vi "DB Tools Create Table If Not Exist.vi"(4 "parameters":T1[](array[typedef]), 5 "use file? (F)":bool, 6 "error in (no error)":errorcluster, 7 "columns":string[](array[string]), 8 "table name":string, 9 "connection reference":T4) -> (0 "error out":errorcluster, 1 "columns out":string[](array[string]), 2 "table name out":string, 3 "connection reference out":T4)   [LabVIEW 2012, in "NI_Database_API_64.lvlib"]
doc: "Creates a new table in the database identified by <B>connection reference</B> if that table does not already exist. The <B>table name</B>, <B>columns</B>, and <B>parameters</B> inputs describe the name of the table, the names of the columns (fields), and the parameter properties of each column, respectively."
uses:
  NI_Database_API_64.lvlib
  Connection.llb/Conn ObjectReference.ctl
  DB Tools Parameter Info.ctl
  DB Tools DataTypes.ctl
  DB Tools Parameter Dir.ctl
  DB Tools Column Info.ctl
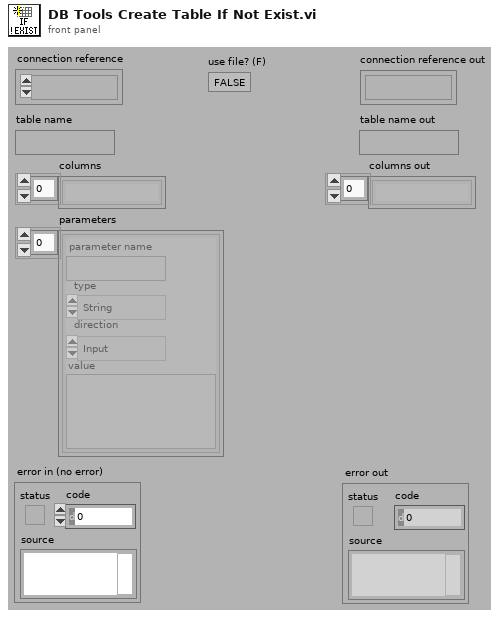
[diagram p1: front panel]
types:
  T1 = typedef "NI_Database_API_64.lvlib/DB Tools Parameter Info.ctl" = cluster{"parameter name":string, "type":T2, "direction":T3, "value":variant}
  T2 = typedef "NI_Database_API_64.lvlib/DB Tools DataTypes.ctl" = enum16{"String", "Long (I32)", "Single (SGL)", "Double (DBL)", "Date/Time", "Binary"}
  T3 = typedef "NI_Database_API_64.lvlib/DB Tools Parameter Dir.ctl" = enum32{"Input", "Output", "Input/Output", "Return Value"}
  T4 = typedef "NI_Database_API_64.lvlib/Conn ObjectReference.ctl" = refnum<k1>
  T5 = typedef "NI_Database_API_64.lvlib/DB Tools Column Info.ctl" = cluster{"column name":string, "data type":T2, "size":i32, "allow null?":bool}
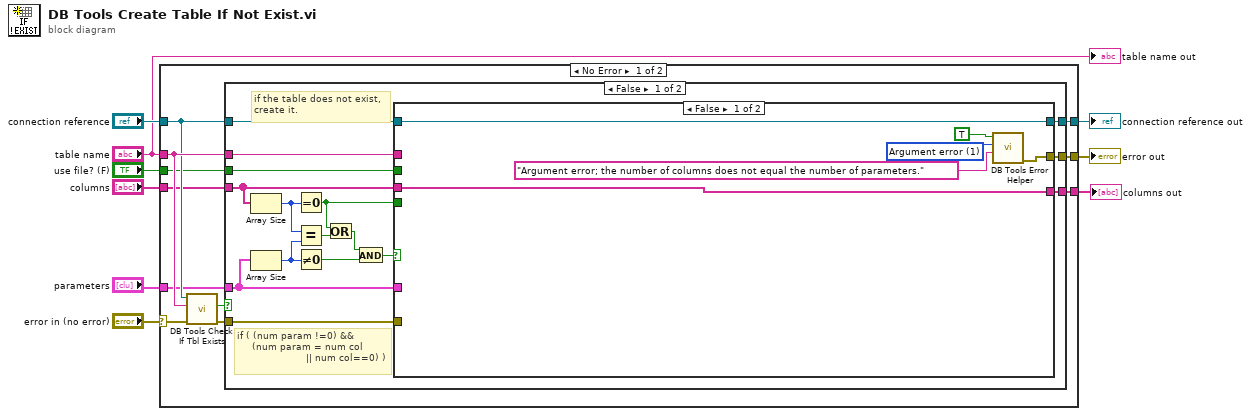
[diagram p0: block diagram]
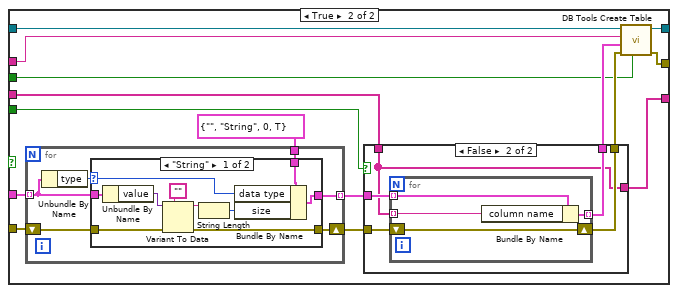
[diagram p2: hidden frame]
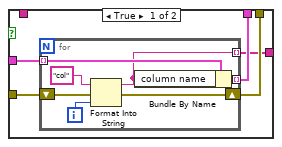
[diagram p3: hidden frame]
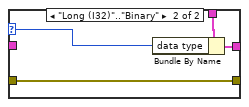
[diagram p4: hidden frame]
diagram:
  n1 = case shown="No Error" "error in (no error)" {
    selector: "error in (no error)" -> [w10 w104]
    tunnel: "connection reference" -> [w15 w103]
    tunnel: "table name" -> [w18 _]
    tunnel: [w17 w104] -> w7
    tunnel: [w16 w103] -> w6
    tunnel: "columns" -> [w14 w102]
    tunnel: "parameters" -> [w12 _]
    tunnel: [w13 w102] -> w3
    tunnel: "use file? (F)" -> [w11 _]
    frame No Error {
      n2 = call "DB Tools Check If Tbl Exists.vi"("error in (no error)"=w10, "table name"=w18, "connection reference"=w15) -> ("error out"=w20:errorcluster, "exists?"=w19:bool)  [unwired: 3 out]
      n3 = case shown="False" w19 {
        tunnel: w20 -> [w26 w101]
        tunnel: w18 -> [w36 _]
        tunnel: [w35 w101] -> w17
        tunnel: [w34 w100] -> w16
        tunnel: w15 -> [w33 w100]
        tunnel: w14 -> [w28 w99]
        tunnel: w12 -> [w22 _]
        tunnel: [w24 w99] -> w13
        tunnel: w11 -> [w21 _]
        frame False {
          # "if ( (num param !=0) &&\n     (num param = num col \n                       || num col==0) )"
          # "if the table does not exist, \ncreate it."
          n4 = Array Size(array=w28) -> (size(s)=w32:i32)
          n5 = Array Size(array=w22) -> (size(s)=w25:i32)
          n6 = Equal To 0?(x=w32) -> (x = 0?=w23:bool)
          n7 = Equal?(x=w32, y=w25) -> (x = y?=w31:bool)
          n8 = Not Equal To 0?(x=w25) -> (x != 0?=w29:bool)
          n9 = Or(x=w23, y=w31) -> (x .or. y?=w30:bool)
          n10 = And(x=w30, y=w29) -> (x .and. y?=w27:bool)
          n11 = case shown="False" w27 {
            tunnel: w36 -> [_ w57]
            tunnel: [w40 w56] -> w35
            tunnel: [w39 w55] -> w34
            tunnel: w33 -> [w39 w54]
            tunnel: w28 -> [w38 w46]
            tunnel: w22 -> [_ w53]
            tunnel: w26 -> [_ w52]
            tunnel: [w38 w44] -> w24
            tunnel: w23 -> [_ w47]
            tunnel: w21 -> [_ w43]
            frame False {
              w42 = 1 items=["No error", "Argument error", "Memory is full", "Out of zone", "End of file", "File already open", "Generic file I/O error", "File not found", "File permission error", "Disk is full", "Duplicate path", "Too many files open", "System feature not enabled", "Resource file not found", "Cannot add resource", "Resource not found", "Image not found", "Image memory error", "Pen does not exist", "Config type invalid", "Config token not found", "Config parse error", "Config memory error", "Bad external code format", "Bad external code offset", "External code not present", "Null window", "Destroy window error", "Null menu", "Print aborted", "Bad print record", "Print driver error", "Windows error during printing", "Memory error during printing", "Print dialog error", "Generic print error", "Invalid device refnum", "Device not found", "Device parameter error", "Device unit error", "Cannot open device", "Device call aborted", "Generic error", "Cancelled by user", "Object ID too low", "Object ID too high", "Object not in heap", "Unknown heap", "Unknown object (invalid DefProc)", "Unknown object (DefProc not in table)", "Message out of range", "Invalid (null) method", "Unknown message", "Manager call not supported", "Bad address", "Network operation in progress", "Network operation timed out", "Connection is busy", "Network attribute not supported", "Network error", "Address in use", "System out of memory", "Connection aborted", "Connection refused", "Not connected", "Already connected", "Connection closed", "Initialization error (interapplication manager)", "Bad occurrence", "Wait on unbound occurrence handler", "Occurrence queue overflow", "Datalog type conflict", "Unused", "Unrecognized type (interapplication manager)", "Memory corrupt", "Failed to make temporary DLL", "Old CIN version", "Drag socket not found", "Failed to load drop-object", "Failed to register OLE object", "Failed to release OLE object", "Format specifier type mismatch", "Unknown format specifier", "Too few format specifiers", "Too many format specifiers", "Scan failed", "Newer CIN version", "Error converting to variant", "Runtime menu error", "Password tampered", "Variant attribute not found", "Incompatible variant data type", "Event data is not available", "Event Store is not present", "Occurrence is not found", "Event Queue is not created", "Event info is not available", "Refnum passed is NULL", "Error retrieving Class GUID", "Error retrieving CoClass GUID", "Error retrieving TypeLib GUID.", "Bad built application magic bytes.", "Specific driver is different from the specific driver associated with the Logical Name.", "There is no session opened to the class driver.", "Max Error", "MAX - Error with config objects", "MAX - Error loading configuration", "MAX - Group not supported"]
              n12 = call "DB Tools Error Helper.vi"("source"="Argument error; the number of columns does not equal the number of parameters.", "code"=w42, "status"=TRUE) -> ("error out"=w40:errorcluster)  [unwired: 1 in, 7 out]
            }
            frame True {
              n13 = for {
                tunnel: w53 -> [w81] mode=indexing
                shift-right: [w82] -> w45
                shift-left: w52 -> [w83]
                tunnel: T5 {"column name"="", "data type"=enum."String", "size"=0, "allow null?"=TRUE} ("column information") -> [w84]
                tunnel: [w80] -> w50 mode=indexing
                n14 = Unbundle By Name(w81) -> ("type"=w79:T2)
                n15 = case shown="\"String\"" w79 {
                  selector: w79 -> [w85 w95]
                  tunnel: [w90 w97] -> w80
                  tunnel: w81 -> [w89 _]
                  tunnel: w84 -> [w86 w96]
                  tunnel: w83 -> [w88 w98]
                  tunnel: [w87 w98] -> w82
                  frame "String" {
                    n16 = Unbundle By Name(w89) -> ("value"=w94:variant)
                    n17 = Variant To Data(error in=w88, type="", Variant=w94) -> (data=w92:string, error out=w87:errorcluster)
                    n18 = String Length(string=w92) -> (length=w91:i32)
                    n19 = Bundle By Name(cluster=w86, "data type"=w85, "size"=w91) -> (w90:T5)
                  }
                  frame "Long (I32)".."Binary" {
                    n20 = Bundle By Name(cluster=w96, "data type"=w95) -> (w97:T5)
                  }
                }
              }
              n21 = case shown="False" w47 {
                tunnel: w50 -> [w62 w74]
                tunnel: [w61 w73] -> w49
                tunnel: [w60 w72] -> w48
                tunnel: w46 -> [_ w70]
                tunnel: w45 -> [w59 w71]
                tunnel: [w58 w70] -> w44
                frame True {
                  n22 = for {
                    shift-right: [w67] -> w60
                    shift-left: w59 -> [w68]
                    tunnel: [w66] -> w61 mode=indexing
                    tunnel: w62 -> [w65] mode=indexing
                    tunnel: [w63] -> w58 mode=indexing
                    i -> [w69]
                    n23 = Format Into String(initial string="col", error in=w68, w69) -> (resulting string=w63:string, error out=w67:errorcluster)  [unwired: 1 in]
                    n24 = Bundle By Name(cluster=w65, "column name"=w63) -> (w66:T5)
                  }
                }
                frame False {
                  n25 = for {
                    shift-right: [w75] -> w72
                    shift-left: w71 -> [w75]
                    tunnel: [w78] -> w73 mode=indexing
                    tunnel: w74 -> [w77] mode=indexing
                    tunnel: w70 -> [w76] mode=indexing
                    n26 = Bundle By Name(cluster=w77, "column name"=w76) -> (w78:T5)
                  }
                }
              }
              n27 = call "DB Tools Create Table.vi"("use file? (F)"=w43, "error in (no error)"=w48, "column information"=w49, "table"=w57, "connection reference"=w54) -> ("error out"=w56:errorcluster, "connection reference out"=w55:T4)  [unwired: 3 out]
            }
          }
        }
        frame True {
          # "if the table exists, the do not create it"
        }
      }
    }
    frame Error {
    }
  }
  "error out" <- w7
  "connection reference out" <- w6
  "columns out" <- w3
  "table name out" <- "table name"
